vi "Start_Trigger.vi"(8 "error in (no error)":errorcluster, 9 "Command_Message_in":T1, 10 "platform":u16(ring) items=["Mac", "PC"], 11 "DAQ_VI":refnum<vi>) -> (0 "error out":errorcluster, 1 "Command_Message_out":T1)   [LabVIEW 2019]
uses:
  Command_Message.ctl
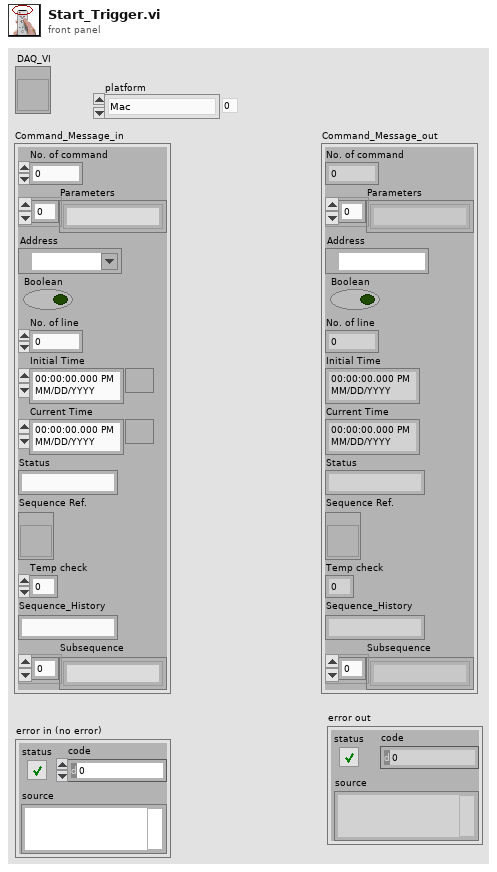
[diagram p1: front panel]
types:
  T1 = typedef "Command_Message.ctl" = cluster{"No. of command":i32, "Parameters":string[], "Address":refnum<visa-resource-name>, "Boolean":bool, "No. of line":i32, "Initial Time":timestamp, "Current Time":timestamp, "Status":string, "Sequence Ref.":refnum<vi>, "Temp check":i32, "Sequence_History":string, "Subsequence":string[]}
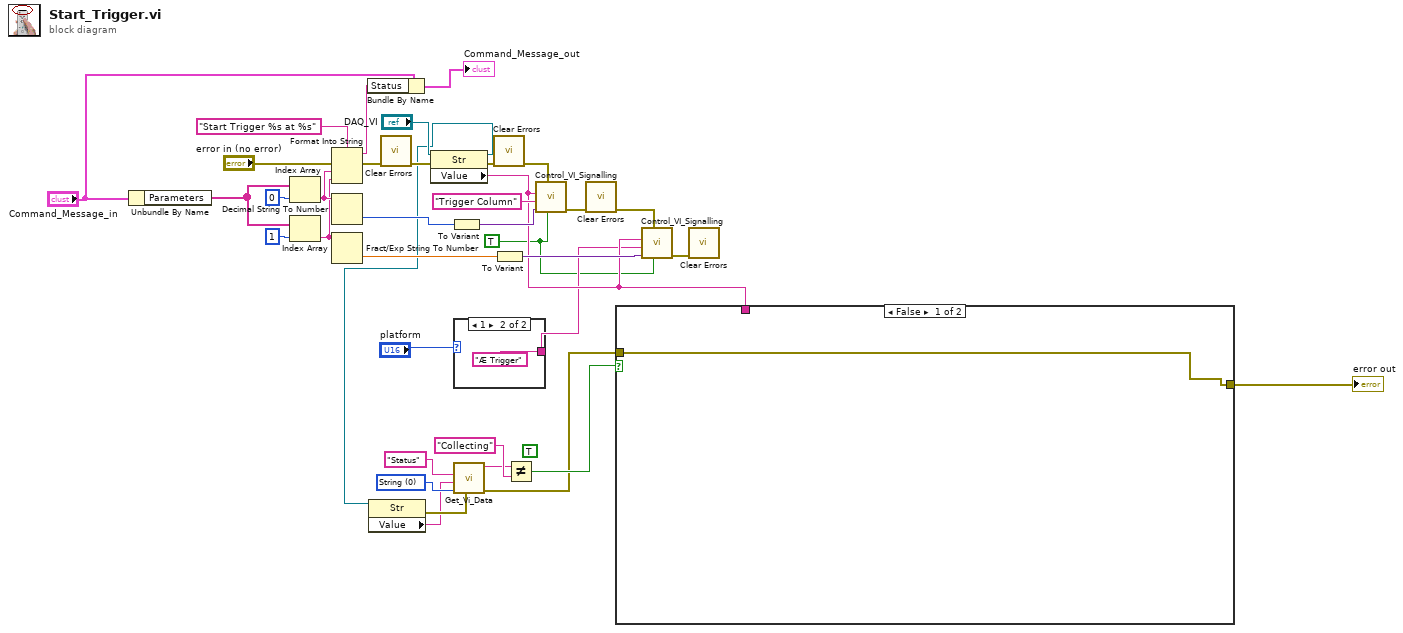
[diagram p0: block diagram]
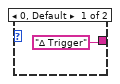
[diagram p2: hidden frame]
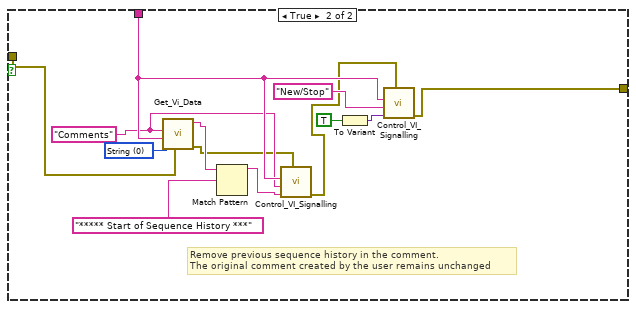
[diagram p3: hidden frame]
diagram:
  w1 = TRUE ("bypass")
  (unwired) TRUE
  w13 = u16 0 items=["String", "Double", "Boolean", "Variant"] ("Data Type")
  n1 = Unbundle By Name("Command_Message_in") -> ("Parameters"=w25:string[])
  n2 = Index Array(array=w25, index=0) -> (element=w28:string)
  n3 = Index Array(array=w25, index=1) -> (element=w27:string)
  n4 = Format Into String(format string="Start Trigger %s at %s", error in="error in (no error)", w28, w27) -> (resulting string=w22:string, error out=w20:errorcluster)  [unwired: 1 in]
  n5 = Decimal String To Number(string=w28) -> (number=w33:i32)  [unwired: 2 in, 1 out]
  n6 = Fract/Exp String To Number(string=w27) -> (number=w31:dbl)  [unwired: 3 in, 1 out]
  n7 = Bundle By Name(cluster="Command_Message_in", "Status"=w22) -> (→"Command_Message_out":T1)
  n8 = call <vilib>:"Clear Errors.vi"("error in (no error)"=w20) -> ("error out"=w19:errorcluster)  [unwired: 5 in, 1 out]
  n9 = property on="Property Node" class="Str"(reference="DAQ_VI", error in=w19) -> (reference out=w6:refnum<vi>, error out=w18:errorcluster, "Value"=w21:string)
  n10 = property on="Property Node" class="Str"(reference=w6) -> (error out=w11:errorcluster, "Value"=w10:string)  [unwired: 1 in, 1 out]
  n11 = To Variant(anything=w33) -> (Variant=w32:variant)
  n12 = case shown="1" "platform" {
    tunnel: ["∆ Trigger" "Æ Trigger"] -> w3
    frame 0, Default {
    }
    frame 1 {
    }
  }
  n13 = call "Get_Vi_Data.vi"("error in (no error) 2"=w11, "Data Type"=w13, "VI name"=w10, "Control Name"="Status") -> ("error out"=w5:errorcluster, "Data (String)"=w8:string)  [unwired: 3 in, 3 out]
  n14 = call <vilib>:"Clear Errors.vi"("error in (no error)"=w18) -> ("error out"=w17:errorcluster)  [unwired: 5 in, 1 out]
  n15 = To Variant(anything=w31) -> (Variant=w30:variant)
  n16 = Not Equal?(x=w8, y="Collecting") -> (x != y?=w7:bool)
  n17 = call "Control_VI_Signalling.vi"("bypass"=w1, "error in (no error)"=w17, "Input Value"=w32, "Control Name"="Trigger Column", "Target VI name"=w21) -> ("error out"=w16:errorcluster)  [unwired: 6 in]
  n18 = call <vilib>:"Clear Errors.vi"("error in (no error)"=w16) -> ("error out"=w15:errorcluster)  [unwired: 5 in, 1 out]
  n19 = case shown="False" w7 {
    tunnel: w21 -> [_ w46]
    tunnel: w5 -> [w40 w49]
    tunnel: [w40 w41] -> w2
    frame False {
    }
    frame True {
      w50 = u16 0 items=["String", "Double", "Boolean", "Variant"] ("Data Type")
      w45 = "Comments" ("Control Name")
      # "Remove previous sequence history in the comment. \nThe original comment created by the user remains unchanged"
      n20 = call "Get_Vi_Data.vi"("error in (no error) 2"=w49, "Data Type"=w50, "VI name"=w46, "Control Name"=w45) -> ("error out"=w43:errorcluster, "Data (String)"=w48:string)  [unwired: 3 in, 3 out]
      n21 = Match Pattern(string=w48, regular expression="***** Start of Sequence History ***" ("Control Name")) -> (before substring=w44:string)  [unwired: 1 in, 3 out]
      n22 = call "Control_VI_Signalling.vi"("error in (no error)"=w43, "Input Value"=w44, "Control Name"=w45, "Target VI name"=w46) -> ("error out"=w42:errorcluster)  [unwired: 7 in]
      n23 = To Variant(anything=TRUE) -> (Variant=w52:variant)
      n24 = call "Control_VI_Signalling.vi"("error in (no error)"=w42, "Input Value"=w52, "Control Name"="New/Stop", "Target VI name"=w46) -> ("error out"=w41:errorcluster)  [unwired: 7 in]
    }
  }
  "error out" <- w2
  n25 = call "Control_VI_Signalling.vi"("bypass"=w1, "error in (no error)"=w15, "Input Value"=w30, "Control Name"=w3, "Target VI name"=w21) -> ("error out"=w14:errorcluster)  [unwired: 6 in]
  n26 = call <vilib>:"Clear Errors.vi"("error in (no error)"=w14) -> ()  [unwired: 5 in, 2 out]
